vi "FlexRIO-DMA-DAQ-5761.vi"(4 "Module Clock":refnum<k21>, 5 "DMATtoHOSTFIFO":refnum<k21>="DMATtoHOST0", 6 "Base Clock":refnum<k21>, 7 "IntermediateFIFO":refnum<k21>="FIFO0", 8 "Enable":bool, 9 "Selected Channels":T1[](array[typedef])=[enum."Empty", enum."Empty", enum."Empty", enum."Empty"], 10 "DMA number":i32, 11 "DMA Control":T2={"DMATtoHOSTNCh"=[4], "DMATtoHOSTFrameType"=[0], "DMATtoHOSTSampleSize"=[2], "DMATtoHOSTBlockNWords"=[4096]}) -> ()   [LabVIEW 2013, in "IRIO.lvlib"]
uses:
  IRIO.lvlib
  ctl/SelectedChannels.ctl
  ctl/AcquisitionStateControl.ctl
  <vilib>/Platform/TimedLoop/XDataNode/timing_clust.ctl
  <vilib>/Platform/TimedLoop/XDataNode/nitl_modes.ctl
  <vilib>/Platform/TimedLoop/XDataNode/wakeup.ctl
  <vilib>/rvi/DataTransferAndStorage/Container/Common/niFpgaContainerExecOnDevCompGetState.vi
  <vilib>/rvi/FIFO/Fifo_Resource/nirvififoEmulationClearFpgaImpl.vi
  <vilib>/rvi/DataTransferAndStorage/Container/Common/niFpgaContainerGetUniqueNameForEmu.vi
  <vilib>/rvi/interface/RandomDataEmulation/nirviRandomDataFPGAFIFO.vi
  <vilib>/rvi/interface/RandomDataEmulation/niFpgaRandomDataHandleErrors.vi
  <vilib>/rvi/eio/common/nirviEmuReportErrorAndStop.vi
  <vilib>/rvi/Emulation/niFpgaSctlEmulationGetInTimedLoop.vi
  <vilib>/rvi/Emulation/niFpgaEmulationReportErrorSimple.vi
  <vilib>/rvi/Emulation/niFpgaGetClockAttributes.vi
  <vilib>/rvi/Emulation/niFpgaCriticalErrorInLSC.vi
  <vilib>/rvi/FIFO/Fifo_Resource/nirvififoEmulationGetNumberOfElementsToReadFpgaImpl.vi
  <vilib>/rvi/FIFO/Fifo_Resource/nirvififoEmulationReadFpgaImpl.vi
  <vilib>/rvi/FIFO/Fifo_Resource/nirvififoEmulationWriteFpgaImpl.vi
  common/GlobalReg.vi
  <vilib>/rvi/DataTransferAndStorage/Container/XNode/niFpgaContainer.xnode
  <vilib>/rvi/FIFO/Fifo_Resource/niFpgaFifoEmulationRefIn.vi
  <vilib>/Platform/TimedLoop/XDataNode/XDataNode.xnode
  <vilib>/rvi/interface/RandomDataEmulation/nirviRandomDataFpgaReadWriteTemplate.vi
  <vilib>/Platform/TimedLoop/XDataNode/XDNodeRunTimeDep.lvlib
panel:
  in  "Enum":T1
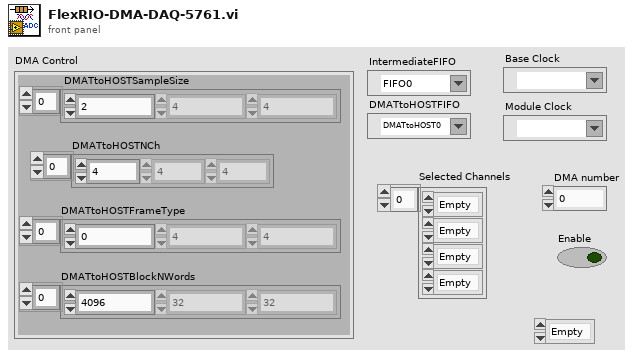
[diagram p1: front panel]
types:
  T1 = typedef "IRIO.lvlib/SelectedChannels.ctl" = enum16{"Empty", "AI0", "AI1", "AI2", "AI3", "SignalGenerator0", "SignalGenerator1", "DDCA_PORT0", "DDCA_PORT1", "DDCA_PORT2", "DDCB_PORT0", "DDCB_PORT1", "DDCB_PORT2"}
  T2 = cluster{"DMATtoHOSTNCh":u16[], "DMATtoHOSTFrameType":u8[], "DMATtoHOSTSampleSize":u8[], "DMATtoHOSTBlockNWords":u16[]}
  T3 = typedef "IRIO.lvlib/AcquisitionStateControl.ctl" = enum16{"Idle", "Acq"}
  T4 = typedef "XDNodeRunTimeDep.lvlib/timing_clust.ctl" = cluster{"Expected End [f-1]":u64, "Actual End [f-1]":u64, "Finished Late? [f-1]":bool, "Expected End [i-1]":u64, "Actual End [i-1]":u64, "Finished Late? [i-1]":bool, "Expected Start [i]":u64, "Actual Start [i]":u64, "Expected Start [f]":u64, "Actual Start [f]":u64, "Source Name":string, "Structure Name":string, "Period":i64, "Deadline":i64, "Offset":i64, "Start":i64, "Priority":i32, "Timeout":i32, "Mode":T5, "Wakeup Reason":T6, "Error":errorcluster, "Source Type":string, "Secondary Source Type":string, "Global End Time":u64, "Global Start Time":u64, "Frame Duration":u64, "Iteration Duration":u64, "Assigned CPU":i32, "I/O Scan Engine Mode":u32}
  T5 = typedef "XDNodeRunTimeDep.lvlib/nitl_modes.ctl" = enum32{"No Change", "Process missed periods, maintain original phase", "Discard missed periods, maintain original phase", "Process missed periods, ignore original phase", "Discard missed periods, ignore original phase"}
  T6 = typedef "XDNodeRunTimeDep.lvlib/wakeup.ctl" = enum32{"Normal", "Aborted", "Asynchronous wakeup", "Timing source error", "Timed loop error", "Timeout"}
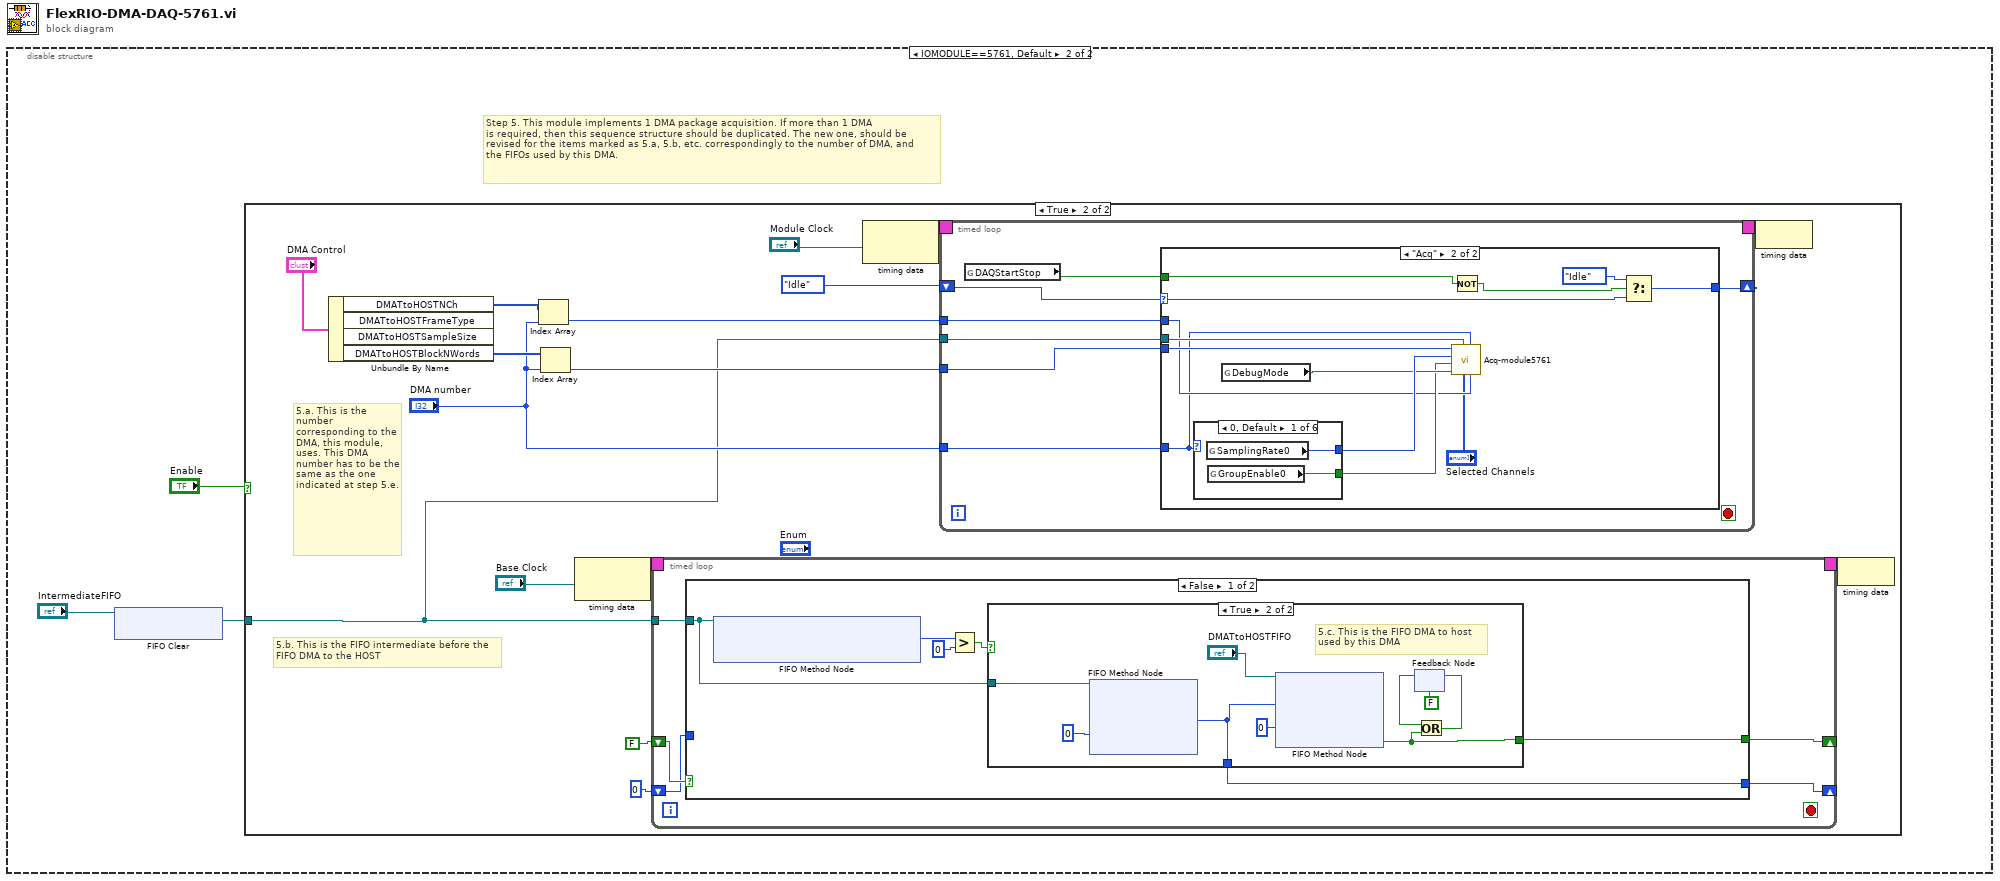
[diagram p0: block diagram]
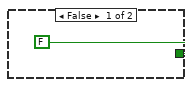
[diagram p4: hidden frame]
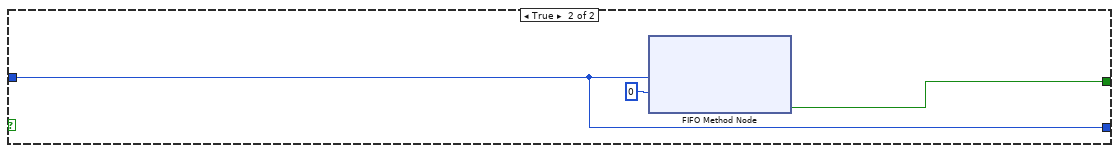
[diagram p5: hidden frame]
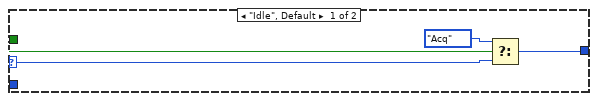
[diagram p6: hidden frame]
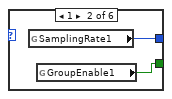
[diagram p7: hidden frame]
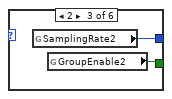
[diagram p8: hidden frame]
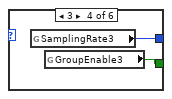
[diagram p9: hidden frame]
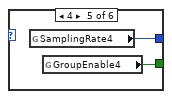
[diagram p10: hidden frame]
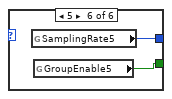
[diagram p11: hidden frame]
diagram:
  n1 = disable-structure shown="IOMODULE==5761, Default" {
    frame condition #0 {
    }
    frame condition #1 (active) {
      # "Step 5. This module implements 1 DMA package acquisition. If more than 1 DMA \nis required, then this sequence structure should be duplicated. The new one, should be \nrevised for the items marked as 5.a, 5.b, etc. correspondingly to the number of DMA, and \nthe FIFOs used by this DMA."
      n2 = xnode ("FIFO Clear")("FIFO In"="IntermediateFIFO") -> ("FIFO Out"=w1:refnum<k21>)
      n3 = case shown="True" "Enable" {
        tunnel: w1 -> [_ w4]
        frame False {
        }
        frame True {
          # "5.b. This is the FIFO intermediate before the \nFIFO DMA to the HOST"
          # "5.a. This is the number corresponding to the \nDMA, this module, uses. This DMA \nnumber has to be the same as the one indicated at step 5.e."
          n4 = Unbundle By Name("DMA Control") -> ("DMATtoHOSTNCh"=w10:u16[], "DMATtoHOSTBlockNWords"=w12:u16[])  [unwired: 2 out]
          n5 = Index Array(array=w10, index="DMA number") -> (element=w9:u16)
          n6 = Index Array(array=w12, index="DMA number") -> (element=w11:u16)
          n7 = node-c288("Base Clock") -> (w17:T4)
          n8 = timed-loop {
            timing: w17 -> [_]
            timing-out: [_] -> w16
            shift-right: [w24] -> _
            shift-left: FALSE ("Timed Out?") -> [w23]
            shift-right: [w22] -> _
            shift-left: u64 0 -> [w21]
            tunnel: w4 -> [w20]
            stop <- _ stop-if-true
            n9 = case shown="False" w23 {
              tunnel: [w27 w42] -> w24
              tunnel: [w26 w41] -> w22
              tunnel: w21 -> [_ w41]
              tunnel: w20 -> [w25 _]
              frame False {
                n10 = xnode ("FIFO Method Node")("FIFO In"=w25) -> ("Number of Elements to Read"=w30:u32)  [unwired: 1 out]
                n11 = Greater?(x=w30, y=u32 0) -> (0:w28:bool)
                n12 = case shown="True" w28 {
                  tunnel: [FALSE ("Timed Out?") w37] -> w27
                  tunnel: [_ w38] -> w26
                  tunnel: w25 -> [_ w33]
                  frame False {
                  }
                  frame True {
                    # "5.c. This is the FIFO DMA to host \nused by this DMA"
                    n13 = xnode ("FIFO Method Node")("Timeout"=0, "FIFO In"=w33) -> ("Element"=w38:u64)  [unwired: 2 out]
                    n14 = xnode ("FIFO Method Node")("Element"=w38, "Timeout"=0, "FIFO In"="DMATtoHOSTFIFO") -> ("Timed Out?"=w37:bool)  [unwired: 1 out]
                    n15 = feedback #1(FALSE) -> (w36:bool)
                    n16 = Or(x=w36, y=w37) -> (x .or. y?=w35:bool)
                    n17 = feedback-in #1(w35) -> ()
                  }
                }
              }
              frame True {
                n18 = xnode ("FIFO Method Node")("Element"=w41, "Timeout"=0) -> ("Timed Out?"=w42:bool)  [unwired: 1 in, 1 out]
              }
            }
          }
          n19 = node-c288("Module Clock") -> (w19:T4)
          n20 = timed-loop {
            timing: w19 -> [_]
            timing-out: [_] -> w18
            shift-right: [w56] -> _
            shift-left: AcquisitionStateControl."Idle" ("Enum") -> [w51]
            tunnel: "DMA number" -> [w54]
            tunnel: w9 -> [w53]
            tunnel: w4 -> [w52]
            tunnel: w11 -> [w50]
            stop <- _ stop-if-true
            n21 = global read "GlobalReg.vi" "DAQStartStop"() -> (w55:bool)
            n22 = case shown="\"Acq\"" w51 {
              selector: w51 -> [w58 w72]
              tunnel: w55 -> [w60 w69]
              tunnel: [w57 w71] -> w56
              tunnel: w54 -> [_ w62]
              tunnel: w53 -> [_ w63]
              tunnel: w52 -> [_ w68]
              tunnel: w50 -> [_ w64]
              frame "Idle", Default {
                n23 = Select(t=AcquisitionStateControl."Acq" ("Enum"), s=w60, f=w58) -> (s? t:f=w57:T3)
              }
              frame "Acq" {
                n24 = case shown="0, Default" w62 {
                  tunnel: [w75 w77 w79 w81 w83 w85] -> w67
                  tunnel: [w74 w76 w78 w80 w82 w84] -> w65
                  frame 0, Default {
                    n25 = global read "GlobalReg.vi" "SamplingRate0"() -> (w75:u16)
                    n26 = global read "GlobalReg.vi" "GroupEnable0"() -> (w74:bool)
                  }
                  frame 1 {
                    n27 = global read "GlobalReg.vi" "SamplingRate1"() -> (w77:u16)
                    n28 = global read "GlobalReg.vi" "GroupEnable1"() -> (w76:bool)
                  }
                  frame 2 {
                    n29 = global read "GlobalReg.vi" "SamplingRate2"() -> (w79:u16)
                    n30 = global read "GlobalReg.vi" "GroupEnable2"() -> (w78:bool)
                  }
                  frame 3 {
                    n31 = global read "GlobalReg.vi" "SamplingRate3"() -> (w81:u16)
                    n32 = global read "GlobalReg.vi" "GroupEnable3"() -> (w80:bool)
                  }
                  frame 4 {
                    n33 = global read "GlobalReg.vi" "SamplingRate4"() -> (w83:u16)
                    n34 = global read "GlobalReg.vi" "GroupEnable4"() -> (w82:bool)
                  }
                  frame 5 {
                    n35 = global read "GlobalReg.vi" "SamplingRate5"() -> (w85:u16)
                    n36 = global read "GlobalReg.vi" "GroupEnable5"() -> (w84:bool)
                  }
                }
                n37 = global read "GlobalReg.vi" "DebugMode"() -> (w66:bool)
                n38 = call "Acq-module5761.vi"("NumChannels"=w63, "DMA number"=w62, "Selected Channels"="Selected Channels", "IntermediateFIFO"=w68, "DebugActivation"=w66, "GroupEnableN"=w65, "SamplingRateN(DecimationFactor)"=w67, "DMATtoHOSTBlockNWords"=w64) -> ()  [unwired: 4 in]
                n39 = Not(x=w69) -> (.not. x?=w70:bool)
                n40 = Select(t=AcquisitionStateControl."Idle" ("Enum"), s=w70, f=w72) -> (s? t:f=w71:T3)
              }
            }
          }
          n41 = node-c288(w18) -> ()
          n42 = node-c288(w16) -> ()
        }
      }
    }
  }
